vi "Host.vi"() -> ()   [LabVIEW 2018]
uses:
  <instrlib>/niDCPower/nidcpower.llb/niDCPower Measurement Type.ctl
panel:
  in  "VDD_PLL_selcur":dbl=0.01 caption="current limit" format="%_6p"
  out "VDD_PLL":i32
  out "VDD_PLL":bool
  in  "RD_selcur":dbl=0.01 caption="current limit" format="%_6p"
  out "RD":i32
  out "RD":bool
  in  "A3PE_selcur":dbl=0.2 caption="current limit" format="%_6p"
  out "A3PE":i32
  out "A3PE":bool
  in  "VDD_RS_selcur":dbl=0.2 caption="current limit" format="%_6p"
  out "VDD_RS":i32
  out "VDD_RS":bool
  in  "VDD_PLL, V":dbl=5.0 caption="voltage level" format="%_6p"
  in  "VDD_PLL_curlim, A":dbl=0.1 caption="current limit" format="%_6p"
  out "VDD_PLL_cur, A":dbl caption="measurement" format="%_6g"
  out "VDD_PLL Chart":dbl(graph)=-0.002263378745703706 caption="Waveform Chart 5"
  in  "RD, V":dbl=5.0 caption="voltage level" format="%_6p"
  in  "RD_curlim, A":dbl=0.1 caption="current limit" format="%_6p"
  out "RD_cur, A":dbl caption="measurement" format="%_6g"
  out "RD Chart":dbl(graph)=0.0390164550609864 caption="Waveform Chart 5"
  in  "A3PE, V":dbl=5.0 caption="voltage level" format="%_6p"
  in  "A3PE_curlim, A":dbl=0.3 caption="current limit" format="%_6p"
  out "A3PE_cur, A":dbl caption="measurement" format="%_6g"
  out "A3PE Chart":dbl(graph)=-0.007994936055928669 caption="Waveform Chart 5"
  in  "ИОС":refnum<k15>="PXI1Slot6" caption="instrument handle"
  in  "RD/VDD_PLL":refnum<k15>="PXI1Slot5" caption="instrument handle"
  in  "ИОС":bool
  in  "ИОС, V":dbl=5.0 caption="voltage level" format="%_6p"
  in  "ИОС_curlim, A":dbl=0.1 caption="current limit" format="%_6p"
  out "ИОС_cur, A":dbl caption="measurement" format="%_6g"
  out "ИОС Chart":dbl(graph)=0.03241218329386533 caption="Waveform Chart 5"
  in  "Период опроса, мс":u32=1
  out "VDD_RS_cur, A":dbl caption="measurement" format="%_6g"
  out "VDD_RS Chart":dbl(graph)=0.03234747481509968 caption="Waveform Chart 5"
  in  "VDD_RS, V":dbl=5.0 caption="voltage level" format="%_6p"
  in  "VDD_RS_curlim, A":dbl=0.25 caption="current limit" format="%_6p"
  in  "VDD_RS/A3PE":refnum<k15>="PXI1Slot4" caption="instrument handle"
  in  "VDD_A_selcur":dbl=0.4 caption="current limit" format="%_6p"
  out "VDD_A":i32
  out "VDD_A":bool
  out "VDD_A_cur, A":dbl caption="measurement" format="%_6g"
  out "VDD_A Chart":dbl(graph)=-0.000235222149982668
  in  "VDD_A, V":dbl=5.0 caption="voltage level" format="%_6p"
  in  "VDD_A_curlim, A":dbl=0.5 caption="current limit" format="%_6p"
  in  "Стоп":bool
  in  "Питание":bool
  in  "SEL_T, мс":u32=100
  in  "SIM_SEL":bool
  out "SEL":bool
  in  "VDD18_selcur":dbl=0.01 caption="current limit" format="%_6p"
  in  "VDD10_selcur":dbl=0.01 caption="current limit" format="%_6p"
  in  "VDD_LVDS_selcur":dbl=0.1 caption="current limit" format="%_6p"
  out "VDD18":i32
  out "VDD18":bool
  out "VDD10":i32
  out "VDD10":bool
  out "VDD_LVDS":i32
  out "VDD_LVDS":bool
  in  "VDD18, V":dbl=5.0 caption="voltage level" format="%_6p"
  in  "VDD18_curlim, A":dbl=0.4 caption="current limit" format="%_6p"
  in  "VDD10_curlim, A":dbl=0.1 caption="current limit" format="%_6p"
  out "VDD18_cur, A":dbl caption="measurement" format="%_6g"
  out "VDD10_cur, A":dbl caption="measurement" format="%_6g"
  in  "VDD10, V":dbl=5.0 caption="voltage level" format="%_6p"
  in  "VDD_LVDS, V":dbl=5.0 caption="voltage level" format="%_6p"
  in  "VDD_LVDS_curlim, A":dbl=0.3 caption="current limit" format="%_6p"
  out "VDD_LVDS_cur, A":dbl caption="measurement" format="%_6g"
  out "VDD10 Chart":dbl(graph)=-0.0025072983641264367
  out "VDD_LVDS Chart":dbl(graph)=-0.0403673797130392
  out "VDD18 Chart":dbl(graph)=0.17110122624002952 caption="Waveform Chart 5"
  in  "VDD18/VDD10":refnum<k15>="PXI1Slot2" caption="instrument handle"
  in  "VDD_LVDS/VDD_A":refnum<k15>="PXI1Slot3" caption="instrument handle"
  in  "SEL":path=path "C:/VPL/LabView_PRJ/Astrolabia_22003/SEL"
  out "Номер образца":string="0"
  # "Астролябия:\n0.0:\n1: +5V_VDD1,8\n2: GND\n\n0.1:\n3: GND\n4: +5V_VDD1,0\n\n1.0:\n6: +5V_VDD_LVDS\n7: GND\n\n1.1:\n9: +5V_VDD_A\n10: GND\n\n2.0:\n12: +5V_VDD_RS\n13: GND\n\n2.1:\n14: +5V_A3PE\n15: GND\n\n3.0:\n18: +5V_RD\n19: GND\n\n3.1:\n24: +5V_VDD_PLL\n25: GND"
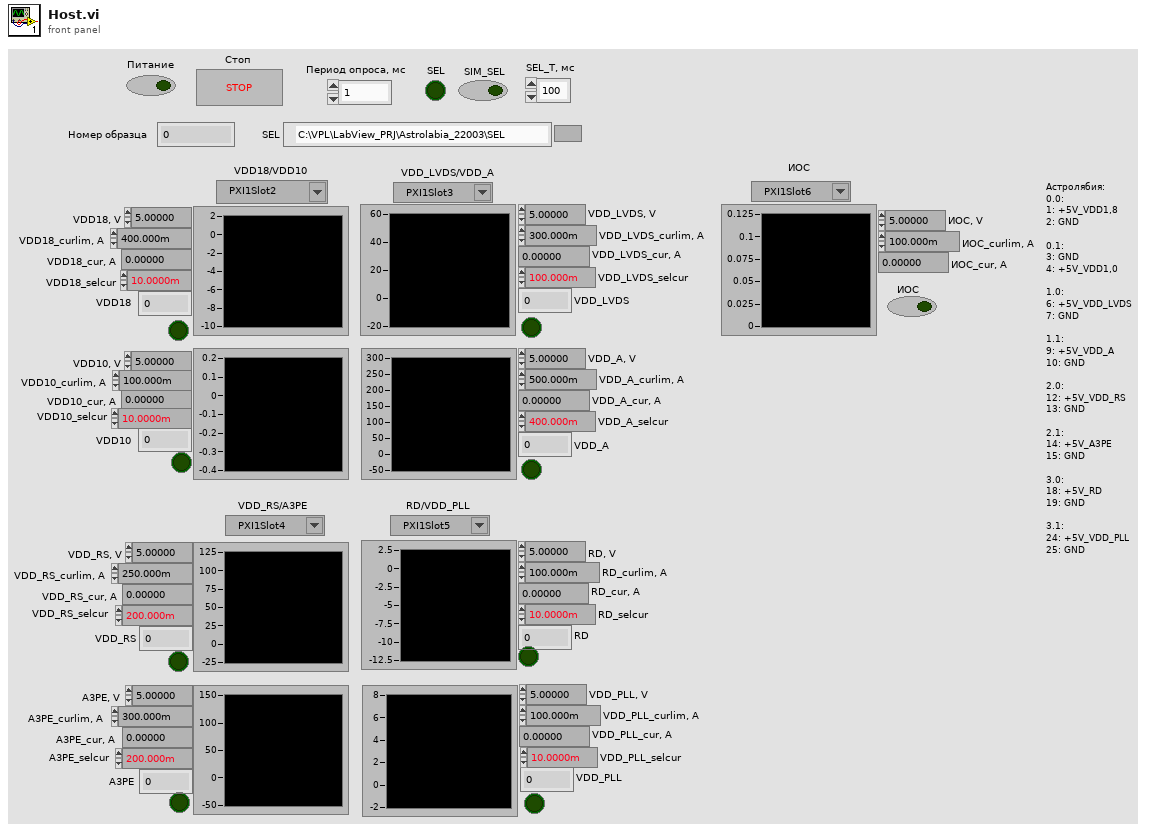
[diagram p1: front panel]
types:
  T1 = enum16{"open", "replace", "create", "open or create", "replace or create", "replace or create with confirmation"}
  T2 = typedef "niDCPower Measurement Type.ctl" = i32
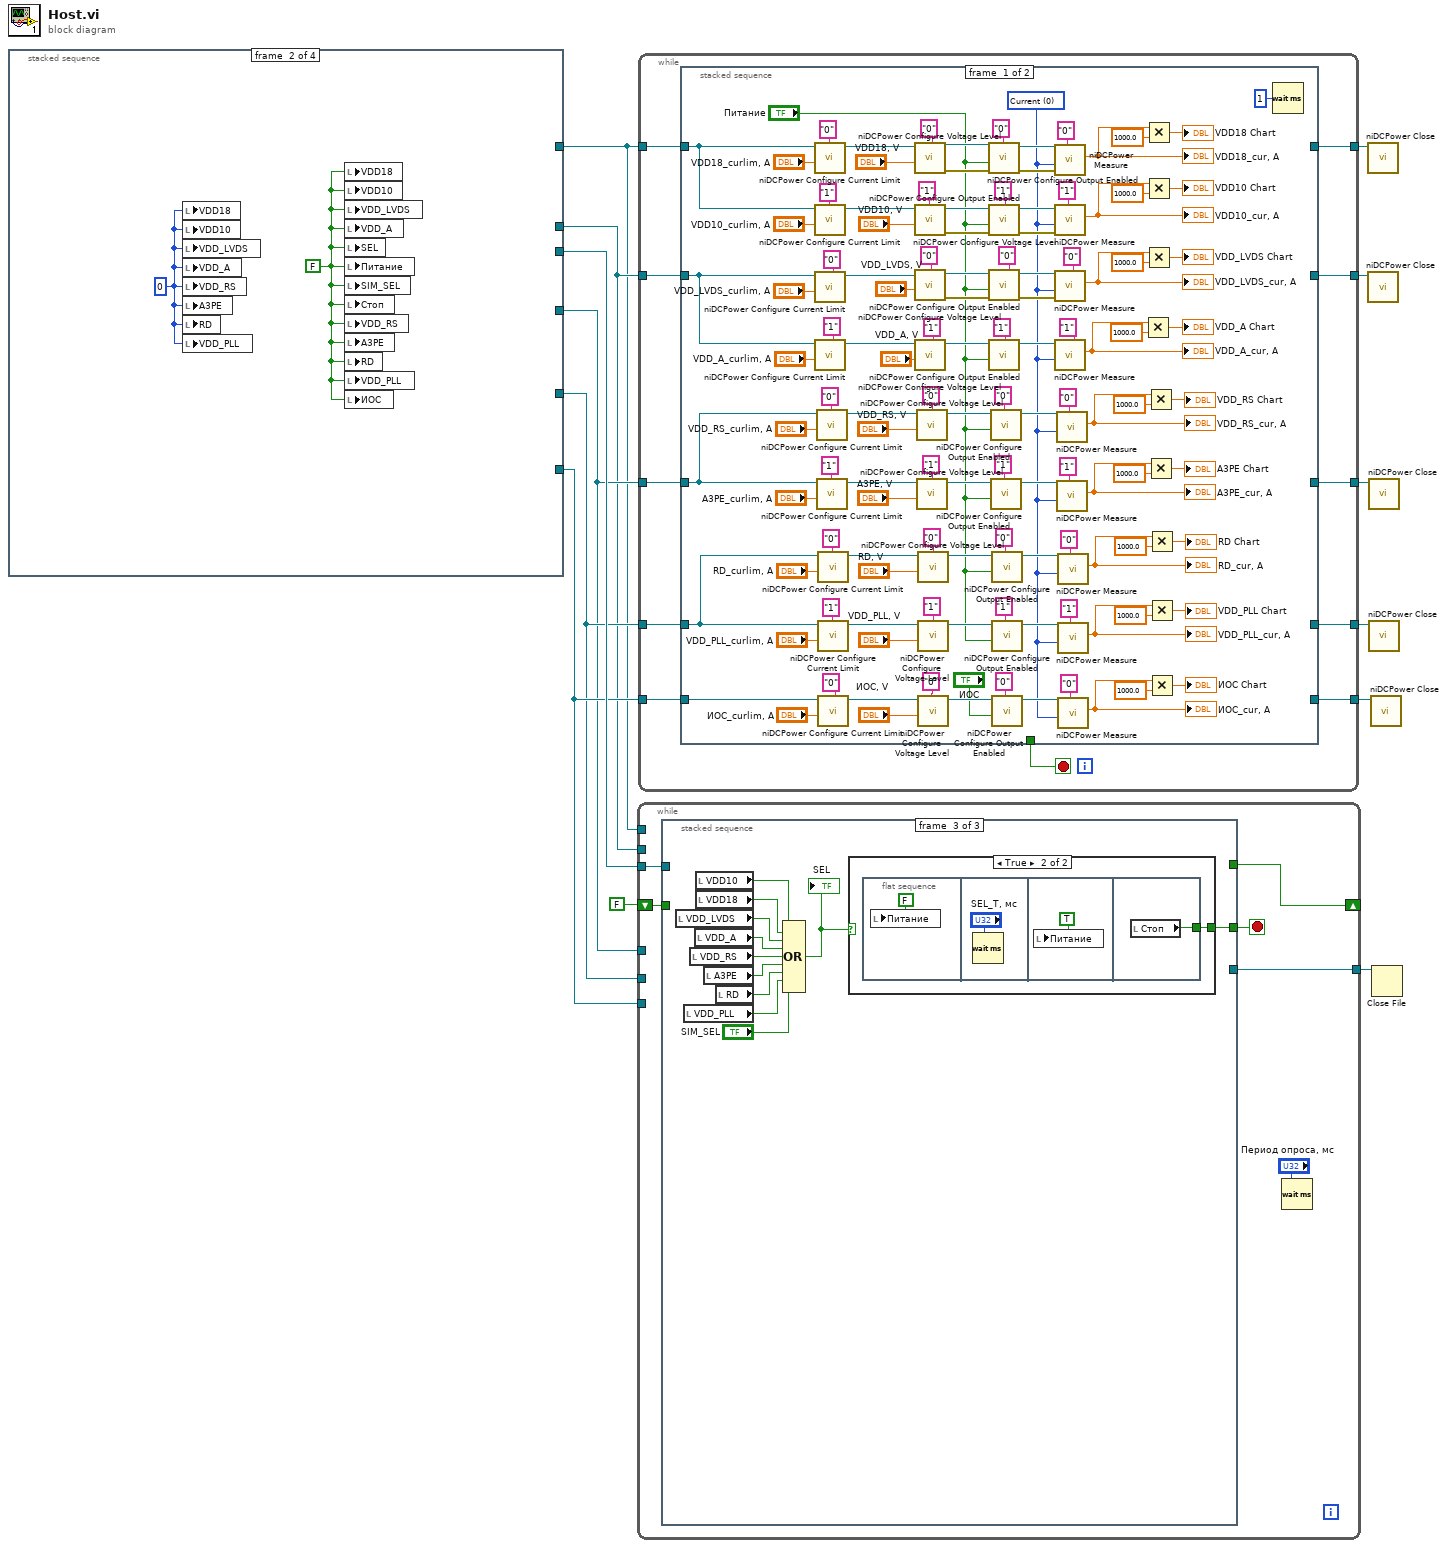
[diagram p0: block diagram]
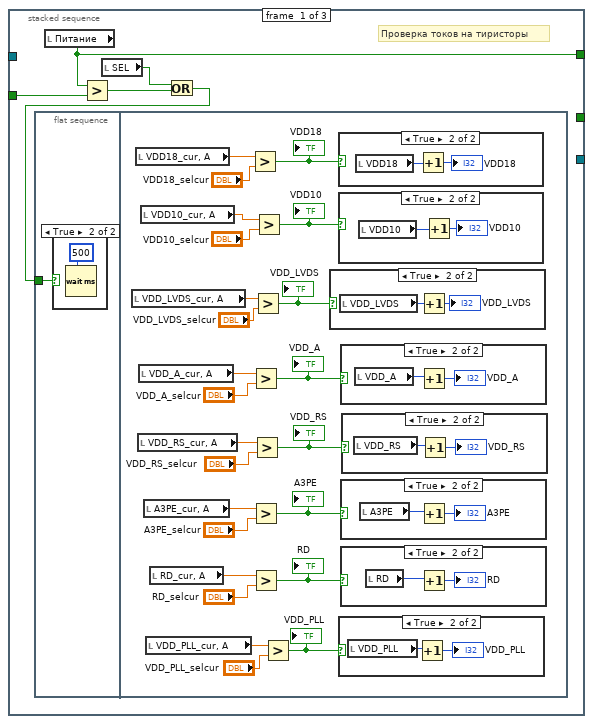
[diagram p2: hidden frame]
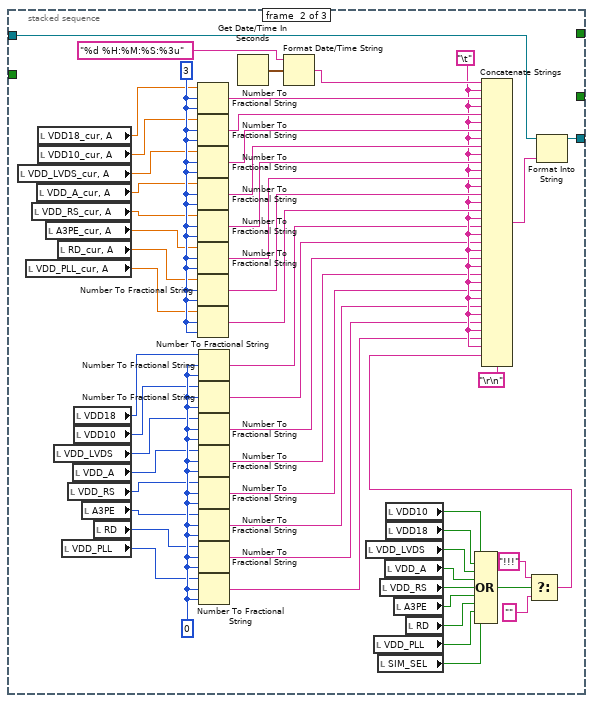
[diagram p12: hidden frame]
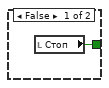
[diagram p13: hidden frame]
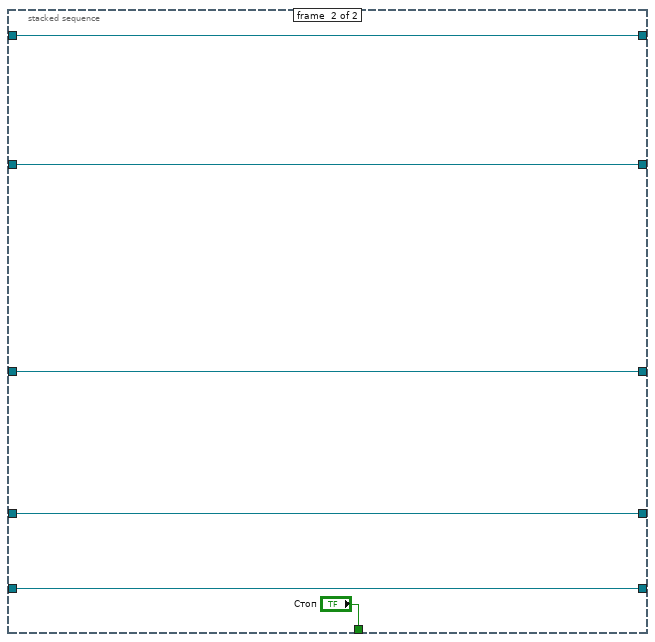
[diagram p14: hidden frame]
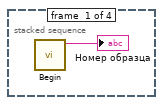
[diagram p15: hidden frame]
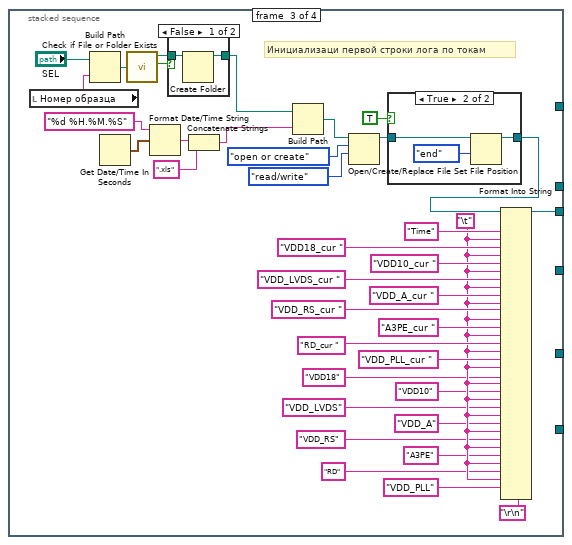
[diagram p16: hidden frame]
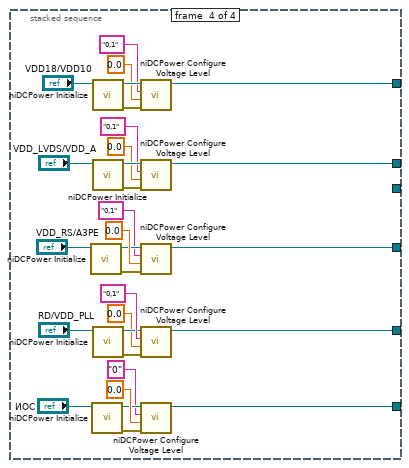
[diagram p19: hidden frame]
diagram:
  n1 = stacked-sequence {
    tunnel: [_ _ _ w80] -> w7
    tunnel: [_ _ _ w79] -> w6
    tunnel: [_ _ w37 _] -> w12
    tunnel: [_ _ _ w73] -> w8
    tunnel: [_ _ _ w62] -> w9
    tunnel: [_ _ _ w61] -> w10
    frame #0 {
      n2 = call "Begin.vi"() -> ("Номер образца 2"=→"Номер образца":string)  [unwired: 11 in]
    }
    frame #1 {
      w16 = 0
      w15 = FALSE
      n3 = local write "VDD18"(w16) -> ()
      n4 = local write "VDD10"(w16) -> ()
      n5 = local write "VDD_LVDS"(w16) -> ()
      n6 = local write "VDD_A"(w16) -> ()
      n7 = local write "VDD_RS"(w16) -> ()
      n8 = local write "A3PE"(w16) -> ()
      n9 = local write "RD"(w16) -> ()
      n10 = local write "VDD_PLL"(w16) -> ()
      n11 = local write "VDD18"(w15) -> ()
      n12 = local write "VDD10"(w15) -> ()
      n13 = local write "VDD_LVDS"(w15) -> ()
      n14 = local write "VDD_A"(w15) -> ()
      n15 = local write "SEL"(w15) -> ()
      n16 = local write "Питание"(w15) -> ()
      n17 = local write "SIM_SEL"(w15) -> ()
      n18 = local write "Стоп"(w15) -> ()
      n19 = local write "VDD_RS"(w15) -> ()
      n20 = local write "A3PE"(w15) -> ()
      n21 = local write "RD"(w15) -> ()
      n22 = local write "VDD_PLL"(w15) -> ()
      n23 = local write "ИОС"(w15) -> ()
    }
    frame #2 {
      w26 = "\t"
      # "Инициализаци первой строки лога по токам"
      n24 = local read "Номер образца"() -> (w49:string)
      n25 = Build Path(base path="SEL", name or relative path=w49) -> (appended path=w51:path)
      n26 = Get Date/Time In Seconds() -> (seconds since 1Jan1904=w44:timestamp)
      n27 = call <vilib>:"Check if File or Folder Exists.vi"("path"=w51) -> ("file or folder exists?"=w52:bool, "dup path"=w53:path)  [unwired: 8 in, 1 out]
      n28 = Format Date/Time String(time format string (%c)="%d %H.%M.%S", seconds (now)=w44) -> (date/time string=w41:string)  [unwired: 1 in]
      n29 = case shown="False" w52 {
        tunnel: w53 -> [w59 w60]
        tunnel: [w58 w60] -> w36
        frame False {
          n30 = Create Folder(path (use dialog)=w59) -> (created path=w58:path)  [unwired: 2 in, 2 out]
        }
        frame True {
        }
      }
      n31 = Concatenate Strings(w41, ".xls" ("string")) -> (w39:string)
      n32 = Build Path(base path=w36, name or relative path=w39) -> (appended path=w42:path)
      n33 = Open/Create/Replace File(file path (use dialog)=w42, operation (0:open)=T1."open or create", access (0:read/write)=enum16{"read/write", "read-only", "write-only"}."read/write") -> (refnum out=w45:refnum<file>)  [unwired: 3 in, 2 out]
      n34 = case shown="True" TRUE {
        tunnel: w45 -> [w54 w57]
        tunnel: [w54 w55] -> w38
        frame False {
        }
        frame True {
          n35 = Set File Position(refnum=w57, from (0:start)=enum16{"start", "end", "current"}."end") -> (refnum out=w55:refnum<file>)  [unwired: 2 in, 1 out]
        }
      }
      n36 = Format Into String(initial string=w38, "Time" ("input 1"), w26, "VDD18_cur " ("input 1"), w26, "VDD10_cur " ("input 1"), w26, "VDD_LVDS_cur " ("input 1"), w26, "VDD_A_cur " ("input 1"), w26, "VDD_RS_cur " ("input 1"), w26, "A3PE_cur " ("input 1"), w26, "RD_cur " ("input 1"), w26, "VDD_PLL_cur " ("input 1"), w26, "VDD18" ("input 1"), w26, "VDD10" ("input 1"), w26, "VDD_LVDS" ("input 1"), w26, "VDD_A" ("input 1"), w26, "VDD_RS" ("input 1"), w26, "A3PE" ("input 1"), w26, "RD" ("input 1"), w26, "VDD_PLL" ("input 1"), "\r\n") -> (resulting string=w37:refnum<file>)  [unwired: 2 in, 1 out]
    }
    frame #3 {
      n37 = call <instrlib>:"niDCPower Initialize.vi"("resource name"="VDD_RS/A3PE") -> ("error out"=w76:errorcluster, "instrument handle out"=w75:refnum<k15>)  [unwired: 3 in, 6 out]
      n38 = call <instrlib>:"niDCPower Initialize.vi"("resource name"="ИОС") -> ("error out"=w65:errorcluster, "instrument handle out"=w64:refnum<k15>)  [unwired: 3 in, 6 out]
      n39 = call <instrlib>:"niDCPower Initialize.vi"("resource name"="VDD18/VDD10") -> ("error out"=w87:errorcluster, "instrument handle out"=w89:refnum<k15>)  [unwired: 3 in, 6 out]
      n40 = call <instrlib>:"niDCPower Initialize.vi"("resource name"="VDD_LVDS/VDD_A") -> ("error out"=w88:errorcluster, "instrument handle out"=w90:refnum<k15>)  [unwired: 3 in, 6 out]
      n41 = call <instrlib>:"niDCPower Initialize.vi"("resource name"="RD/VDD_PLL") -> ("error out"=w70:errorcluster, "instrument handle out"=w71:refnum<k15>)  [unwired: 3 in, 6 out]
      n42 = call <instrlib>:"niDCPower Configure Voltage Level.vi"("error in (no error)"=w87, "voltage level"=0.0, "channel name"="0,1", "instrument handle"=w89) -> ("instrument handle out"=w79:refnum<k15>)  [unwired: 6 in, 1 out]
      n43 = call <instrlib>:"niDCPower Configure Voltage Level.vi"("error in (no error)"=w88, "voltage level"=0.0, "channel name"="0,1", "instrument handle"=w90) -> ("instrument handle out"=w80:refnum<k15>)  [unwired: 6 in, 1 out]
      n44 = call <instrlib>:"niDCPower Configure Voltage Level.vi"("error in (no error)"=w76, "voltage level"=0.0, "channel name"="0,1", "instrument handle"=w75) -> ("instrument handle out"=w73:refnum<k15>)  [unwired: 6 in, 1 out]
      n45 = call <instrlib>:"niDCPower Configure Voltage Level.vi"("error in (no error)"=w70, "voltage level"=0.0, "channel name"="0,1", "instrument handle"=w71) -> ("instrument handle out"=w62:refnum<k15>)  [unwired: 6 in, 1 out]
      n46 = call <instrlib>:"niDCPower Configure Voltage Level.vi"("error in (no error)"=w65, "voltage level"=0.0, "channel name"="0", "instrument handle"=w64) -> ("instrument handle out"=w61:refnum<k15>)  [unwired: 6 in, 1 out]
    }
  }
  n47 = while {
    shift-right: [w96] -> _
    shift-left: FALSE -> [w95]
    tunnel: w12 -> [w94]
    tunnel: [w92] -> w11
    tunnel: w10 -> [_]
    tunnel: w9 -> [_]
    tunnel: w8 -> [_]
    tunnel: w7 -> [_]
    tunnel: w6 -> [_]
    stop <- w93 stop-if-true
    n48 = stacked-sequence {
      tunnel: [w100 _ _] -> w96
      tunnel: w95 -> [w101 _ _]
      tunnel: w94 -> [_ w188 _]
      tunnel: [_ _ w209] -> w93
      tunnel: [_ w186 _] -> w92
      frame #0 {
        # "Проверка токов на тиристоры"
        n49 = flat-sequence {
          tunnel: w97 -> [w102]
          frame #0 {
            n50 = case shown="True" w102 {
              frame False {
              }
              frame True {
                n51 = Wait (ms)(milliseconds to wait=u32 500) -> ()  [unwired: 1 out]
              }
            }
          }
          frame #1 {
            n52 = local read "VDD_LVDS_cur, A"() -> (w119:dbl)
            n53 = local read "VDD18_cur, A"() -> (w121:dbl)
            n54 = local read "VDD_RS_cur, A"() -> (w113:dbl)
            n55 = local read "VDD_A_cur, A"() -> (w118:dbl)
            n56 = local read "VDD10_cur, A"() -> (w120:dbl)
            n57 = local read "A3PE_cur, A"() -> (w112:dbl)
            n58 = local read "VDD_PLL_cur, A"() -> (w106:dbl)
            n59 = local read "RD_cur, A"() -> (w107:dbl)
            n60 = Greater?(x=w121, y="VDD18_selcur") -> (0:w126:bool)
            "VDD18" <- w126
            n61 = Greater?(x=w118, y="VDD_A_selcur") -> (0:w117:bool)
            "VDD_A" <- w117
            n62 = Greater?(x=w112, y="A3PE_selcur") -> (0:w111:bool)
            "A3PE" <- w111
            n63 = Greater?(x=w107, y="RD_selcur") -> (0:w108:bool)
            "RD" <- w108
            n64 = Greater?(x=w113, y="VDD_RS_selcur") -> (0:w114:bool)
            "VDD_RS" <- w114
            n65 = Greater?(x=w119, y="VDD_LVDS_selcur") -> (0:w122:bool)
            "VDD_LVDS" <- w122
            n66 = Greater?(x=w120, y="VDD10_selcur") -> (0:w124:bool)
            "VDD10" <- w124
            n67 = Greater?(x=w106, y="VDD_PLL_selcur") -> (0:w105:bool)
            "VDD_PLL" <- w105
            n68 = case shown="True" w122 {
              frame False {
              }
              frame True {
                n69 = local read "VDD_LVDS"() -> (w139:i32)
                n70 = Increment(x=w139) -> (x+1=→"VDD_LVDS":i32)
              }
            }
            n71 = case shown="True" w126 {
              frame False {
              }
              frame True {
                n72 = local read "VDD18"() -> (w143:i32)
                n73 = Increment(x=w143) -> (x+1=→"VDD18":i32)
              }
            }
            n74 = case shown="True" w124 {
              frame False {
              }
              frame True {
                n75 = local read "VDD10"() -> (w140:i32)
                n76 = Increment(x=w140) -> (x+1=→"VDD10":i32)
              }
            }
            n77 = case shown="True" w105 {
              frame False {
              }
              frame True {
                n78 = local read "VDD_PLL"() -> (w129:i32)
                n79 = Increment(x=w129) -> (x+1=→"VDD_PLL":i32)
              }
            }
            n80 = case shown="True" w117 {
              frame False {
              }
              frame True {
                n81 = local read "VDD_A"() -> (w137:i32)
                n82 = Increment(x=w137) -> (x+1=→"VDD_A":i32)
              }
            }
            n83 = case shown="True" w111 {
              frame False {
              }
              frame True {
                n84 = local read "A3PE"() -> (w133:i32)
                n85 = Increment(x=w133) -> (x+1=→"A3PE":i32)
              }
            }
            n86 = case shown="True" w108 {
              frame False {
              }
              frame True {
                n87 = local read "RD"() -> (w131:i32)
                n88 = Increment(x=w131) -> (x+1=→"RD":i32)
              }
            }
            n89 = case shown="True" w114 {
              frame False {
              }
              frame True {
                n90 = local read "VDD_RS"() -> (w135:i32)
                n91 = Increment(x=w135) -> (x+1=→"VDD_RS":i32)
              }
            }
          }
        }
        n92 = local read "Питание"() -> (w100:bool)
        n93 = Greater?(x=w100, y=w101) -> (0:w99:bool)
        n94 = local read "SEL"() -> (w98:bool)
        n95 = Or(x=w98, y=w99) -> (x .or. y?=w97:bool)
      }
      frame #1 {
        w184 = i16 0 ("width (-)")
        w185 = i16 3 ("width (-)")
        w178 = "\t"
        n96 = local read "VDD_LVDS_cur, A"() -> (w165:dbl)
        n97 = local read "VDD_PLL_cur, A"() -> (w160:dbl)
        n98 = local read "VDD_RS_cur, A"() -> (w163:dbl)
        n99 = local read "VDD_A_cur, A"() -> (w164:dbl)
        n100 = local read "VDD18_cur, A"() -> (w167:dbl)
        n101 = local read "VDD10_cur, A"() -> (w166:dbl)
        n102 = local read "A3PE_cur, A"() -> (w162:dbl)
        n103 = local read "VDD_LVDS"() -> (w157:i32)
        n104 = local read "RD_cur, A"() -> (w161:dbl)
        n105 = local read "VDD_PLL"() -> (w152:i32)
        n106 = local read "VDD_RS"() -> (w155:i32)
        n107 = local read "VDD_A"() -> (w156:i32)
        n108 = local read "VDD18"() -> (w159:i32)
        n109 = local read "VDD10"() -> (w158:i32)
        n110 = local read "A3PE"() -> (w154:i32)
        n111 = local read "RD"() -> (w153:i32)
        n112 = Number To Fractional String(number=w167, width (-)=w185, precision (6)=w185) -> (F-format string=w192:string)  [unwired: 1 in]
        n113 = Number To Fractional String(number=w166, width (-)=w185, precision (6)=w185) -> (F-format string=w191:string)  [unwired: 1 in]
        n114 = Number To Fractional String(number=w165, width (-)=w185, precision (6)=w185) -> (F-format string=w190:string)  [unwired: 1 in]
        n115 = Number To Fractional String(number=w164, width (-)=w185, precision (6)=w185) -> (F-format string=w187:string)  [unwired: 1 in]
        n116 = Number To Fractional String(number=w163, width (-)=w185, precision (6)=w185) -> (F-format string=w182:string)  [unwired: 1 in]
        n117 = Number To Fractional String(number=w162, width (-)=w185, precision (6)=w185) -> (F-format string=w181:string)  [unwired: 1 in]
        n118 = Number To Fractional String(number=w161, width (-)=w185, precision (6)=w185) -> (F-format string=w180:string)  [unwired: 1 in]
        n119 = Number To Fractional String(number=w160, width (-)=w185, precision (6)=w185) -> (F-format string=w179:string)  [unwired: 1 in]
        n120 = Number To Fractional String(number=w159, width (-)=w184, precision (6)=w184) -> (F-format string=w176:string)  [unwired: 1 in]
        n121 = Number To Fractional String(number=w158, width (-)=w184, precision (6)=w184) -> (F-format string=w175:string)  [unwired: 1 in]
        n122 = Number To Fractional String(number=w157, width (-)=w184, precision (6)=w184) -> (F-format string=w174:string)  [unwired: 1 in]
        n123 = Number To Fractional String(number=w156, width (-)=w184, precision (6)=w184) -> (F-format string=w173:string)  [unwired: 1 in]
        n124 = Number To Fractional String(number=w155, width (-)=w184, precision (6)=w184) -> (F-format string=w172:string)  [unwired: 1 in]
        n125 = Number To Fractional String(number=w154, width (-)=w184, precision (6)=w184) -> (F-format string=w171:string)  [unwired: 1 in]
        n126 = Number To Fractional String(number=w153, width (-)=w184, precision (6)=w184) -> (F-format string=w170:string)  [unwired: 1 in]
        n127 = Number To Fractional String(number=w152, width (-)=w184, precision (6)=w184) -> (F-format string=w169:string)  [unwired: 1 in]
        n128 = Get Date/Time In Seconds() -> (seconds since 1Jan1904=w198:timestamp)
        n129 = Format Date/Time String(time format string (%c)="%d %H:%M:%S:%3u", seconds (now)=w198) -> (date/time string=w193:string)  [unwired: 1 in]
        n130 = local read "VDD_LVDS"() -> (w149:bool)
        n131 = local read "VDD_PLL"() -> (w146:bool)
        n132 = local read "SIM_SEL"() -> (w147:bool)
        n133 = local read "VDD_RS"() -> (w183:bool)
        n134 = local read "VDD_A"() -> (w148:bool)
        n135 = local read "VDD10"() -> (w151:bool)
        n136 = local read "VDD18"() -> (w150:bool)
        n137 = local read "A3PE"() -> (w144:bool)
        n138 = local read "RD"() -> (w145:bool)
        n139 = Compound Arithmetic op=OR(w151, w150, w149, w148, w183, w144, w145, w146, w147) -> (w189:bool)
        n140 = Select(t="!!!", s=w189, f="") -> (s? t:f=w168:string)
        n141 = Concatenate Strings(w193, w178, w192, w178, w191, w178, w190, w178, w187, w178, w182, w178, w181, w178, w180, w178, w179, w178, w176, w178, w175, w178, w174, w178, w173, w178, w172, w178, w171, w178, w170, w178, w169, w178, w168, "\r\n") -> (w197:string)
        n142 = Format Into String(initial string=w188, w197) -> (resulting string=w186:refnum<file>)  [unwired: 2 in, 1 out]
      }
      frame #2 {
        n143 = local read "VDD_LVDS"() -> (w203:bool)
        n144 = local read "VDD_PLL"() -> (w201:bool)
        n145 = local read "VDD_RS"() -> (w208:bool)
        n146 = local read "VDD_A"() -> (w202:bool)
        n147 = local read "VDD10"() -> (w206:bool)
        n148 = local read "VDD18"() -> (w204:bool)
        n149 = local read "A3PE"() -> (w199:bool)
        n150 = local read "RD"() -> (w200:bool)
        n151 = Compound Arithmetic op=OR(w206, w204, w203, w202, w208, w199, w200, w201, "SIM_SEL") -> (w207:bool)
        "SEL" <- w207
        n152 = case shown="True" w207 {
          tunnel: [w210 w211] -> w209
          frame False {
            n153 = local read "Стоп"() -> (w210:bool)
          }
          frame True {
            n154 = flat-sequence {
              tunnel: [w215] -> w211
              frame #0 {
                n155 = local write "Питание"(FALSE ("SYS_RESET")) -> ()
              }
              frame #1 {
                n156 = Wait (ms)(milliseconds to wait="SEL_T, мс") -> ()  [unwired: 1 out]
              }
              frame #2 {
                n157 = local write "Питание"(TRUE ("SYS_RESET")) -> ()
              }
              frame #3 {
                n158 = local read "Стоп"() -> (w215:bool)
              }
            }
          }
        }
      }
    }
    n159 = Wait (ms)(milliseconds to wait="Период опроса, мс") -> ()  [unwired: 1 out]
  }
  n160 = while {
    tunnel: w6 -> [w226]
    tunnel: w10 -> [w223]
    tunnel: w9 -> [w222]
    tunnel: w8 -> [w224]
    tunnel: w7 -> [w225]
    tunnel: [w221] -> w5
    tunnel: [w220] -> w4
    tunnel: [w219] -> w3
    tunnel: [w218] -> w2
    tunnel: [w217] -> w1
    stop <- w216 stop-if-true
    n161 = stacked-sequence {
      tunnel: w223 -> [w269 w351]
      tunnel: w222 -> [w231 w352]
      tunnel: w224 -> [w230 w353]
      tunnel: w225 -> [w229 w354]
      tunnel: w226 -> [w228 w355]
      tunnel: [_ w355] -> w221
      tunnel: [_ w354] -> w220
      tunnel: [_ w353] -> w219
      tunnel: [_ w352] -> w218
      tunnel: [_ w351] -> w217
      tunnel: [_ "Стоп"] -> w216
      frame #0 {
        w232 = T2 0 items=["Current", "Voltage"] ("measurement type")
        n162 = call <instrlib>:"niDCPower Configure Current Limit.vi"("current limit"="VDD18_curlim, A", "channel name"="0", "instrument handle"=w228) -> ("instrument handle out"=w338:refnum<k15>)  [unwired: 7 in, 1 out]
        n163 = call <instrlib>:"niDCPower Configure Current Limit.vi"("current limit"="VDD10_curlim, A", "channel name"="1", "instrument handle"=w228) -> ("instrument handle out"=w339:refnum<k15>)  [unwired: 7 in, 1 out]
        n164 = call <instrlib>:"niDCPower Configure Current Limit.vi"("current limit"="VDD_LVDS_curlim, A", "channel name"="0", "instrument handle"=w229) -> ("instrument handle out"=w321:refnum<k15>)  [unwired: 7 in, 1 out]
        n165 = call <instrlib>:"niDCPower Configure Current Limit.vi"("current limit"="VDD_A_curlim, A", "channel name"="1", "instrument handle"=w229) -> ("instrument handle out"=w301:refnum<k15>)  [unwired: 7 in, 1 out]
        n166 = call <instrlib>:"niDCPower Configure Current Limit.vi"("current limit"="VDD_RS_curlim, A", "channel name"="0", "instrument handle"=w230) -> ("instrument handle out"=w285:refnum<k15>)  [unwired: 7 in, 1 out]
        n167 = call <instrlib>:"niDCPower Configure Current Limit.vi"("current limit"="A3PE_curlim, A", "channel name"="1", "instrument handle"=w230) -> ("instrument handle out"=w259:refnum<k15>)  [unwired: 7 in, 1 out]
        n168 = call <instrlib>:"niDCPower Configure Current Limit.vi"("current limit"="RD_curlim, A", "channel name"="0", "instrument handle"=w231) -> ("instrument handle out"=w254:refnum<k15>)  [unwired: 7 in, 1 out]
        n169 = call <instrlib>:"niDCPower Configure Current Limit.vi"("current limit"="VDD_PLL_curlim, A", "channel name"="1", "instrument handle"=w231) -> ("instrument handle out"=w235:refnum<k15>)  [unwired: 7 in, 1 out]
        n170 = call <instrlib>:"niDCPower Configure Current Limit.vi"("current limit"="ИОС_curlim, A", "channel name"="0", "instrument handle"=w269) -> ("instrument handle out"=w290:refnum<k15>)  [unwired: 7 in, 1 out]
        n171 = call <instrlib>:"niDCPower Configure Voltage Level.vi"("voltage level"="VDD18, V", "channel name"="0", "instrument handle"=w338) -> ("error out"=w331:errorcluster, "instrument handle out"=w334:refnum<k15>)  [unwired: 7 in]
        n172 = call <instrlib>:"niDCPower Configure Voltage Level.vi"("voltage level"="VDD10, V", "channel name"="1", "instrument handle"=w339) -> ("error out"=w332:errorcluster, "instrument handle out"=w333:refnum<k15>)  [unwired: 7 in]
        n173 = call <instrlib>:"niDCPower Configure Voltage Level.vi"("voltage level"="VDD_LVDS, V", "channel name"="0", "instrument handle"=w321) -> ("error out"=w325:errorcluster, "instrument handle out"=w326:refnum<k15>)  [unwired: 7 in]
        n174 = call <instrlib>:"niDCPower Configure Voltage Level.vi"("voltage level"="VDD_A, V", "channel name"="1", "instrument handle"=w301) -> ("instrument handle out"=w299:refnum<k15>)  [unwired: 7 in, 1 out]
        n175 = call <instrlib>:"niDCPower Configure Voltage Level.vi"("voltage level"="VDD_RS, V", "channel name"="0", "instrument handle"=w285) -> ("instrument handle out"=w284:refnum<k15>)  [unwired: 7 in, 1 out]
        n176 = call <instrlib>:"niDCPower Configure Voltage Level.vi"("voltage level"="A3PE, V", "channel name"="1", "instrument handle"=w259) -> ("instrument handle out"=w260:refnum<k15>)  [unwired: 7 in, 1 out]
        n177 = call <instrlib>:"niDCPower Configure Voltage Level.vi"("voltage level"="RD, V", "channel name"="0", "instrument handle"=w254) -> ("instrument handle out"=w253:refnum<k15>)  [unwired: 7 in, 1 out]
        n178 = call <instrlib>:"niDCPower Configure Voltage Level.vi"("voltage level"="VDD_PLL, V", "channel name"="1", "instrument handle"=w235) -> ("instrument handle out"=w236:refnum<k15>)  [unwired: 7 in, 1 out]
        n179 = call <instrlib>:"niDCPower Configure Voltage Level.vi"("voltage level"="ИОС, V", "channel name"="0", "instrument handle"=w290) -> ("instrument handle out"=w291:refnum<k15>)  [unwired: 7 in, 1 out]
        n180 = call <instrlib>:"niDCPower Configure Output Enabled.vi"("error in (no error)"=w331, "output enabled"="Питание", "channel name"="0", "instrument handle"=w334) -> ("error out"=w343:errorcluster, "instrument handle out"=w342:refnum<k15>)  [unwired: 6 in]
        n181 = call <instrlib>:"niDCPower Configure Output Enabled.vi"("error in (no error)"=w332, "output enabled"="Питание", "channel name"="1", "instrument handle"=w333) -> ("error out"=w344:errorcluster, "instrument handle out"=w345:refnum<k15>)  [unwired: 6 in]
        n182 = call <instrlib>:"niDCPower Configure Output Enabled.vi"("error in (no error)"=w325, "output enabled"="Питание", "channel name"="0", "instrument handle"=w326) -> ("error out"=w317:errorcluster, "instrument handle out"=w318:refnum<k15>)  [unwired: 6 in]
        n183 = call <instrlib>:"niDCPower Configure Output Enabled.vi"("output enabled"="Питание", "channel name"="1", "instrument handle"=w299) -> ("instrument handle out"=w297:refnum<k15>)  [unwired: 7 in, 1 out]
        n184 = call <instrlib>:"niDCPower Configure Output Enabled.vi"("output enabled"="Питание", "channel name"="0", "instrument handle"=w284) -> ("instrument handle out"=w283:refnum<k15>)  [unwired: 7 in, 1 out]
        n185 = call <instrlib>:"niDCPower Configure Output Enabled.vi"("output enabled"="Питание", "channel name"="1", "instrument handle"=w260) -> ("instrument handle out"=w261:refnum<k15>)  [unwired: 7 in, 1 out]
        n186 = call <instrlib>:"niDCPower Configure Output Enabled.vi"("output enabled"="Питание", "channel name"="0", "instrument handle"=w253) -> ("instrument handle out"=w252:refnum<k15>)  [unwired: 7 in, 1 out]
        n187 = call <instrlib>:"niDCPower Configure Output Enabled.vi"("output enabled"="Питание", "channel name"="1", "instrument handle"=w236) -> ("instrument handle out"=w237:refnum<k15>)  [unwired: 7 in, 1 out]
        n188 = call <instrlib>:"niDCPower Configure Output Enabled.vi"("output enabled"="ИОС", "channel name"="0", "instrument handle"=w291) -> ("instrument handle out"=w292:refnum<k15>)  [unwired: 7 in, 1 out]
        n189 = call <instrlib>:"niDCPower Measure.vi"("error in (no error)"=w343, "measurement type"=w232, "channel name"="0", "instrument handle"=w342) -> ("measurement"=w310:dbl)  [unwired: 5 in, 2 out]
        "VDD18_cur, A" <- w310
        n190 = call <instrlib>:"niDCPower Measure.vi"("error in (no error)"=w344, "measurement type"=w232, "channel name"="1", "instrument handle"=w345) -> ("measurement"=w313:dbl)  [unwired: 5 in, 2 out]
        "VDD10_cur, A" <- w313
        n191 = call <instrlib>:"niDCPower Measure.vi"("error in (no error)"=w317, "measurement type"=w232, "channel name"="0", "instrument handle"=w318) -> ("measurement"=w311:dbl)  [unwired: 5 in, 2 out]
        "VDD_LVDS_cur, A" <- w311
        n192 = call <instrlib>:"niDCPower Measure.vi"("measurement type"=w232, "channel name"="1", "instrument handle"=w297) -> ("measurement"=w295:dbl)  [unwired: 6 in, 2 out]
        "VDD_A_cur, A" <- w295
        n193 = call <instrlib>:"niDCPower Measure.vi"("measurement type"=w232, "channel name"="0", "instrument handle"=w283) -> ("measurement"=w282:dbl)  [unwired: 6 in, 2 out]
        "VDD_RS_cur, A" <- w282
        n194 = call <instrlib>:"niDCPower Measure.vi"("measurement type"=w232, "channel name"="1", "instrument handle"=w261) -> ("measurement"=w262:dbl)  [unwired: 6 in, 2 out]
        "A3PE_cur, A" <- w262
        n195 = call <instrlib>:"niDCPower Measure.vi"("measurement type"=w232, "channel name"="0", "instrument handle"=w252) -> ("measurement"=w251:dbl)  [unwired: 6 in, 2 out]
        "RD_cur, A" <- w251
        n196 = call <instrlib>:"niDCPower Measure.vi"("measurement type"=w232, "channel name"="1", "instrument handle"=w237) -> ("measurement"=w238:dbl)  [unwired: 6 in, 2 out]
        "VDD_PLL_cur, A" <- w238
        n197 = call <instrlib>:"niDCPower Measure.vi"("measurement type"=w232, "channel name"="0", "instrument handle"=w292) -> ("measurement"=w293:dbl)  [unwired: 6 in, 2 out]
        "ИОС_cur, A" <- w293
        n198 = Multiply(x=w295, y=1000.0) -> (x*y=→"VDD_A Chart":dbl)
        n199 = Multiply(x=w310, y=1000.0) -> (x*y=→"VDD18 Chart":dbl)
        n200 = Multiply(x=w313, y=1000.0) -> (x*y=→"VDD10 Chart":dbl)
        n201 = Multiply(x=w311, y=1000.0) -> (x*y=→"VDD_LVDS Chart":dbl)
        n202 = Multiply(x=w282, y=1000.0) -> (x*y=→"VDD_RS Chart":dbl)
        n203 = Multiply(x=w262, y=1000.0) -> (x*y=→"A3PE Chart":dbl)
        n204 = Multiply(x=w251, y=1000.0) -> (x*y=→"RD Chart":dbl)
        n205 = Multiply(x=w238, y=1000.0) -> (x*y=→"VDD_PLL Chart":dbl)
        n206 = Multiply(x=w293, y=1000.0) -> (x*y=→"ИОС Chart":dbl)
        n207 = Wait (ms)(milliseconds to wait=u32 1) -> ()  [unwired: 1 out]
      }
      frame #1 {
      }
    }
  }
  n208 = call <instrlib>:"niDCPower Close.vi"("instrument handle"=w5) -> ()  [unwired: 10 in, 1 out]
  n209 = call <instrlib>:"niDCPower Close.vi"("instrument handle"=w4) -> ()  [unwired: 10 in, 1 out]
  n210 = call <instrlib>:"niDCPower Close.vi"("instrument handle"=w3) -> ()  [unwired: 10 in, 1 out]
  n211 = call <instrlib>:"niDCPower Close.vi"("instrument handle"=w2) -> ()  [unwired: 10 in, 1 out]
  n212 = call <instrlib>:"niDCPower Close.vi"("instrument handle"=w1) -> ()  [unwired: 10 in, 1 out]
  n213 = Close File(refnum=w11) -> ()  [unwired: 1 in, 2 out]
